vi "Unit Test for Angle to Position.vi"() -> ()   [LabVIEW 2017]
panel:
  out "Backarm Angle\nDegrees 1":dbl format="%.2f"
  out "Forearm Angle\nDegrees 1":dbl format="%.2f"
  out "Backarm Angle\nDegrees 2":dbl format="%.2f"
  out "Forearm Angle\nDegrees 2":dbl format="%.2f"
  out "Count":i32
  out "Backarm Angle":dbl
  out "Forearm Angle":dbl
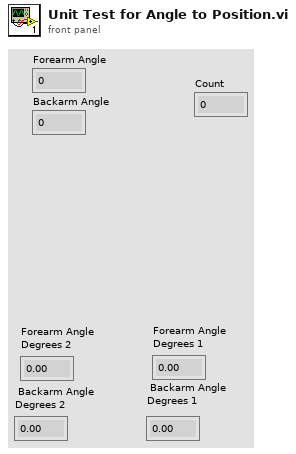
[diagram p1: front panel]
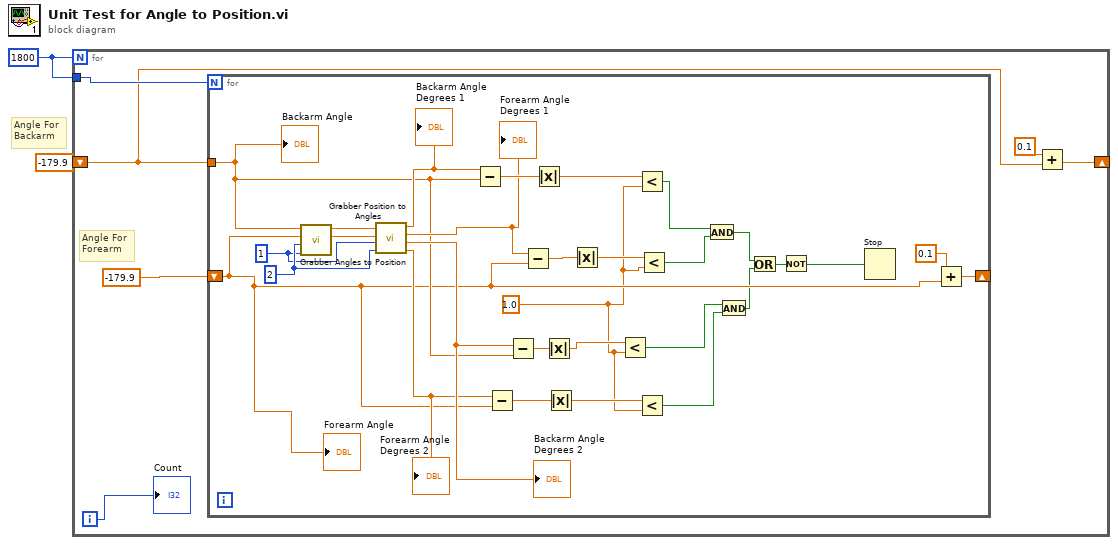
[diagram p0: block diagram]
diagram:
  w2 = 1800
  # "Angle For\nBackarm"
  n1 = for {
    N: w2 -> [_]
    tunnel: w2 -> [w8]
    shift-right: [w5] -> _
    shift-left: -179.9 -> [w6]
    i -> [w3]
    # "Angle For\nForearm"
    n2 = for {
      N: w8 -> [_]
      tunnel: w6 -> [w23]
      shift-right: [w35] -> _
      shift-left: -179.9 -> [w18]
      w10 = 2
      w17 = 1.0
      w9 = 1
      n3 = call "Grabber Angles to Position.vi"("Forerm Length"=w9, "Backarm Length"=w10, "Forearm Angle Degrees"=w18, "Backarm Angle Degrees"=w23) -> ("Y Final"=w36:dbl, "X Final"=w37:dbl)  [unwired: 6 in]
      n4 = call "Grabber Position to Angles.vi"("Backarm Length"=w10, "Forearm Length"=w9, "Y Initial"=w36, "X Initial"=w37) -> ("Forearm Angle\nDegrees 2"=w19:dbl, "Backarm Angle\nDegrees 2"=w24:dbl, "Forearm Angle\nDegrees 1"=w26:dbl, "Backarm Angle\nDegrees 1"=w30:dbl)  [unwired: 4 in]
      "Forearm Angle\nDegrees 2" <- w19
      "Backarm Angle\nDegrees 2" <- w24
      "Forearm Angle\nDegrees 1" <- w26
      "Backarm Angle\nDegrees 1" <- w30
      n5 = Subtract(x=w30, y=w23) -> (x-y=w31:dbl)
      n6 = Subtract(x=w19, y=w18) -> (x-y=w21:dbl)
      n7 = Subtract(x=w24, y=w23) -> (x-y=w25:dbl)
      n8 = Subtract(x=w26, y=w18) -> (x-y=w28:dbl)
      n9 = Absolute Value(x=w31) -> (abs(x)=w29:dbl)
      n10 = Absolute Value(x=w25) -> (abs(x)=w22:dbl)
      n11 = Absolute Value(x=w21) -> (abs(x)=w20:dbl)
      n12 = Absolute Value(x=w28) -> (abs(x)=w27:dbl)
      n13 = Less?(x=w22, y=w17) -> (x < y?=w14:bool)
      n14 = Less?(x=w29, y=w17) -> (x < y?=w15:bool)
      n15 = Less?(x=w20, y=w17) -> (x < y?=w11:bool)
      n16 = Less?(x=w27, y=w17) -> (x < y?=w16:bool)
      n17 = And(x=w15, y=w16) -> (x .and. y?=w12:bool)
      n18 = And(x=w14, y=w11) -> (x .and. y?=w13:bool)
      n19 = Or(x=w12, y=w13) -> (x .or. y?=w33:bool)
      n20 = Not(x=w33) -> (.not. x?=w32:bool)
      n21 = Stop(stop? (T)=w32) -> ()
      n22 = Add(x=0.1, y=w18) -> (x+y=w35:dbl)
      "Forearm Angle" <- w18
      "Backarm Angle" <- w23
    }
    n23 = Add(x=0.1, y=w6) -> (x+y=w5:dbl)
    "Count" <- w3
  }
